vi "MGCC_EnergyMgmt_EMS.vi"() -> ()   [LabVIEW 2016]
uses:
  <vilib>/imath/engines/lvmath2/RunTimeEngine/IndexRead/NIMS V(S).vi
  <vilib>/imath/engines/lvmath2/RunTimeEngine/ErrorHandling/NIMS_Create Error From Enums.vi
  <vilib>/imath/engines/lvmath2/RunTimeEngine/BuiltInFunctions/tril/NIMS_tril.vi
  <vilib>/imath/engines/lvmath2/RunTimeEngine/BuiltInFunctions/double/NIMS_double.vi
  <vilib>/imath/engines/lvmath2/RunTimeEngine/NodeEndStatement/NIMS_NodeEndStatement_Output.vi
  <vilib>/imath/engines/lvmath2/RunTimeEngine/ErrorHandling/NIMS_Finalize Error.vi
  <vilib>/imath/engines/lvmath2/RunTimeEngine/RowToken/NIMS_RowToken_M_CV.vi
  <vilib>/imathl/engines/lvmath/Functions/Error Handling/Create Error.vi
  <vilib>/imath/engines/lvmath/Functions/Error Handling/MergeErrorsWrapper.vi
  <vilib>/imath/engines/lvmath2/RunTimeEngine/IndexRead/NIMS V(R2).vi
  <vilib>/imath/engines/lvmath2/RunTimeEngine/MatrixToken/NIMS_MatrixToken_M_M.vi
  <vilib>/imath/engines/lvmath2/RunTimeEngine/BuiltInFunctions/fmin_lp/NIMS_fmin_lp.vi
  <vilib>/imath/engines/lvmath2/RunTimeEngine/RowToken/NIMS_RowToken_M_M.vi
  <vilib>/imath/engines/lvmath2/RunTimeEngine/BuiltInFunctions/length/NIMS_length(GV).vi
  <vilib>/imath/engines/lvmath2/RunTimeEngine/BuiltInFunctions/eye/NIMS_M=eye(I32).vi
  <vilib>/imath/engines/lvmath2/RunTimeEngine/MatrixToken/NIMS_MatrixToken_M_SorCV.vi
  <vilib>/imath/engines/lvmath2/RunTimeEngine/BuiltInFunctions/is_nan/NIMS_is_nan.vi
  <vilib>/ErrorRing/Error Ring.xnode
  <vilib>/Utility/error.llb/Error Cluster From Error Code.vi
  <vilib>/imath/engines/lvmath2/RunTimeEngine/BuiltInFunctions/max/1 input/NIMS_max(RV).vi
  <vilib>/imath/engines/lvmath2/RunTimeEngine/IndexRead/NIMS V(R3).vi
  <vilib>/imath/engines/lvmath2/RunTimeSupport/NIMS_Get Scalar_w Error.vi
  <vilib>/imath/engines/lvmath2/RunTimeEngine/MatrixToken/NIMS_MatrixToken_M_RV.vi
  <vilib>/imath/engines/lvmath2/RunTimeEngine/BuiltInFunctions/mean/NIMS_RS=mean(RV,I32).vi
  <vilib>/imath/engines/lvmath2/RunTimeEngine/RowToken/NIMS_RowToken_CV_CV.vi
  <vilib>/imath/engines/lvmath2/RunTimeEngine/IndexRead/NIMS M(S,$).vi
  <vilib>/imath/engines/lvmath2/RunTimeEngine/RangeToken/NIMS_Range_R2 - Integer.vi
  <vilib>/imath/engines/lvmath2/RunTimeEngine/ArithmeticOperatorToken/NIMS_ArithmeticOperator_multmx(RV,M)-internal.vi
  <vilib>/imath/engines/lvmath2/RunTimeEngine/BuiltInFunctions/ones/NIMS_V=ones(I32,I32).vi
  <vilib>/imath/engines/lvmath2/RunTimeEngine/ArithmeticOperatorToken/NIMS_ArithmeticOperator_plus.vi
  <vilib>/imath/engines/lvmath2/RunTimeEngine/ArithmeticOperatorToken/NIMS_ArithmeticOperator_minus.vi
  <vilib>/imath/engines/lvmath2/RunTimeEngine/IndexReplace/NIMS V(S)=S.vi
  <vilib>/imath/engines/lvmath2/RunTimeEngine/CommandStatement/MC_CommandStatement_break.vi
  <vilib>/imath/engines/lvmath2/RunTimeEngine/BuiltInFunctions/min/1 input/NIMS_min(RV).vi
  <vilib>/imath/engines/lvmath2/RunTimeEngine/BuiltInFunctions/abs/NIMS_abs(signed).vi
  <vilib>/imath/engines/lvmath2/RunTimeEngine/BuiltInFunctions/findnz/NIMS_[1o]_findnz(GRowV).vi
  <vilib>/imath/engines/lvmath2/RunTimeEngine/BuiltInFunctions/is_empty/NIMS_is_empty(GV).vi
  <vilib>/imath/engines/lvmath2/RunTimeEngine/IndexRead/NIMS M($,V).vi
  <vilib>/imath/engines/lvmath2/RunTimeEngine/IndexReplace/NIMS M($,S)=M.vi
  <vilib>/imath/engines/lvmath2/RunTimeEngine/IndexRead/NIMS M($,S).vi
  <vilib>/imath/engines/lvmath2/RunTimeEngine/ArithmeticOperatorToken/NIMS_ArithmeticOperator_multmx(RV,CV)-internal.vi
panel:
  out "error out ISD1":errorcluster
  out "P_batt1 2":dbl[](array[numeric])
  out "P_batt 3":dbl[](array[numeric])
  out "P_pv1":dbl[](array[numeric])
  out "P_pv":dbl[](array[numeric])
  out "error out 3":errorcluster
  out "L9":dbl[](array[numeric])
  out "L8":dbl[](array[numeric])
  out "L7":dbl[](array[numeric])
  out "L5":dbl[](array[numeric])
  out "L4":dbl[](array[numeric])
  out "L3":dbl[](array[numeric])
  out "L2":dbl[](array[numeric])
  out "L11":dbl[](array[numeric])
  out "L10":dbl[](array[numeric])
  out "P_batt1":dbl[](array[numeric])
  out "HIS8":dbl[](array[numeric])
  out "HIS7":dbl[](array[numeric])
  out "HIS5":dbl[](array[numeric])
  out "HIS4":dbl[](array[numeric])
  out "HIS3":dbl[](array[numeric])
  out "HIS2":dbl[](array[numeric])
  out "HIS9":dbl[](array[numeric])
  out "HIS11":dbl[](array[numeric])
  out "HIS10":dbl[](array[numeric])
  out "P_batt 2":dbl[](array[numeric])
  out "f_MGCC_PVFcst_FcstPV 2":dbl[](array[numeric])
  out "BESS-SOC 2":dbl
  out "Ld 2":dbl[](array[numeric])
  out "error out 2":errorcluster
  out "P_batt":dbl[](array[numeric])
  out "f_MGCC_PVFcst_FcstPV":dbl[](array[numeric])
  out "BESS-SOC":dbl
  out "Ld":dbl[](array[numeric])
  out "error out":errorcluster
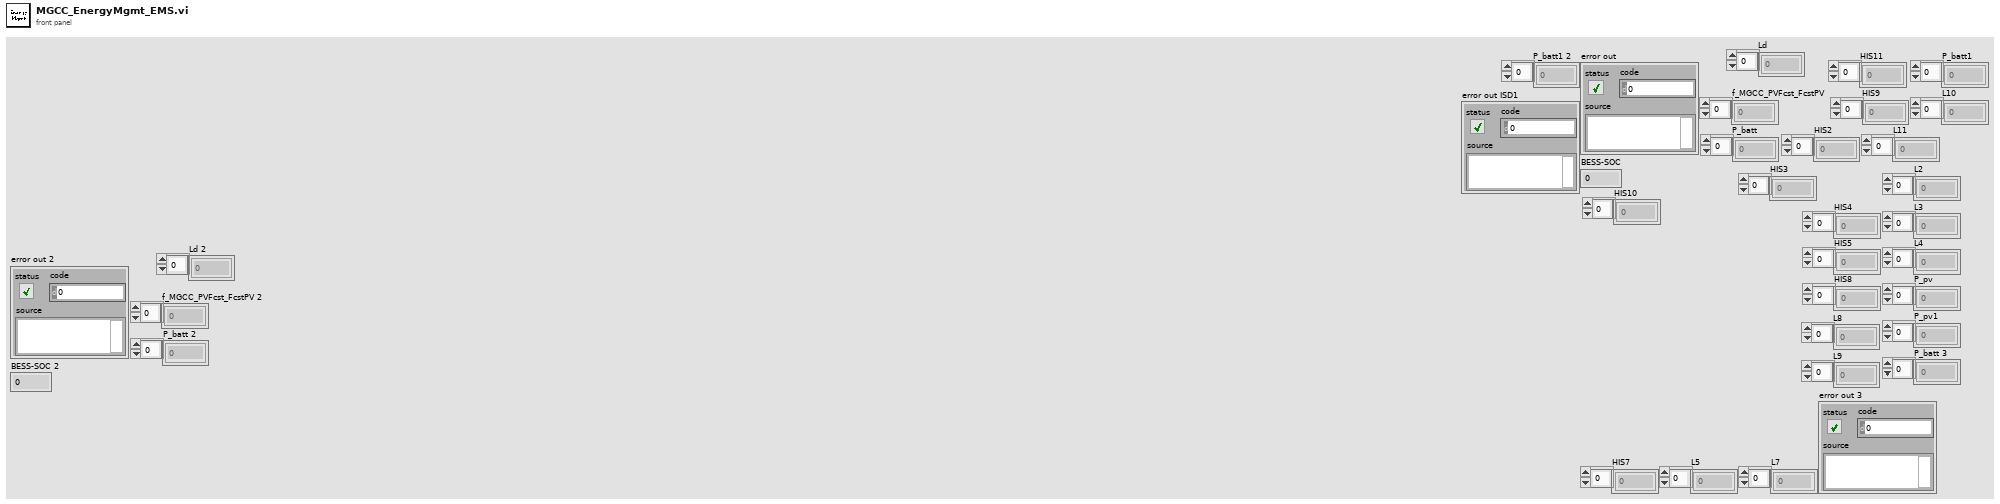
[diagram p1: front panel]
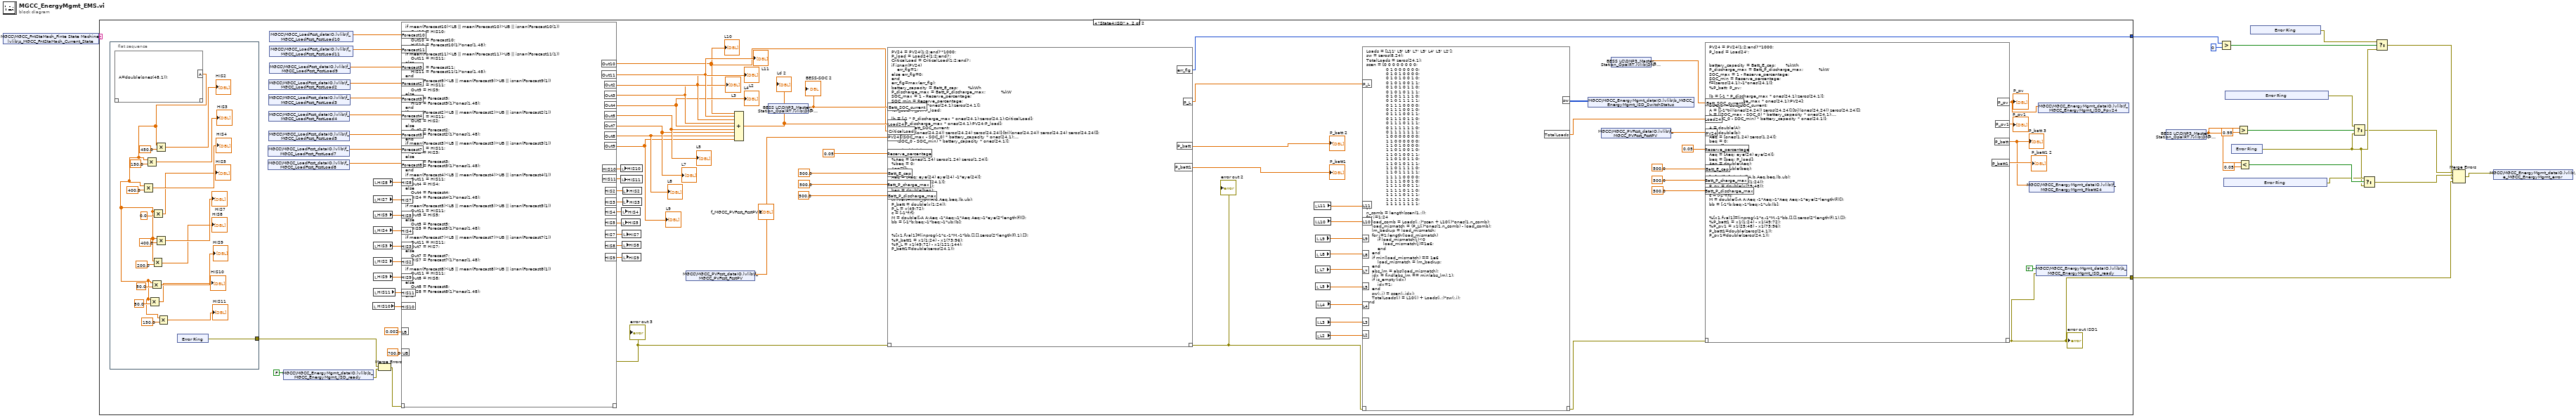
[diagram p0: block diagram]
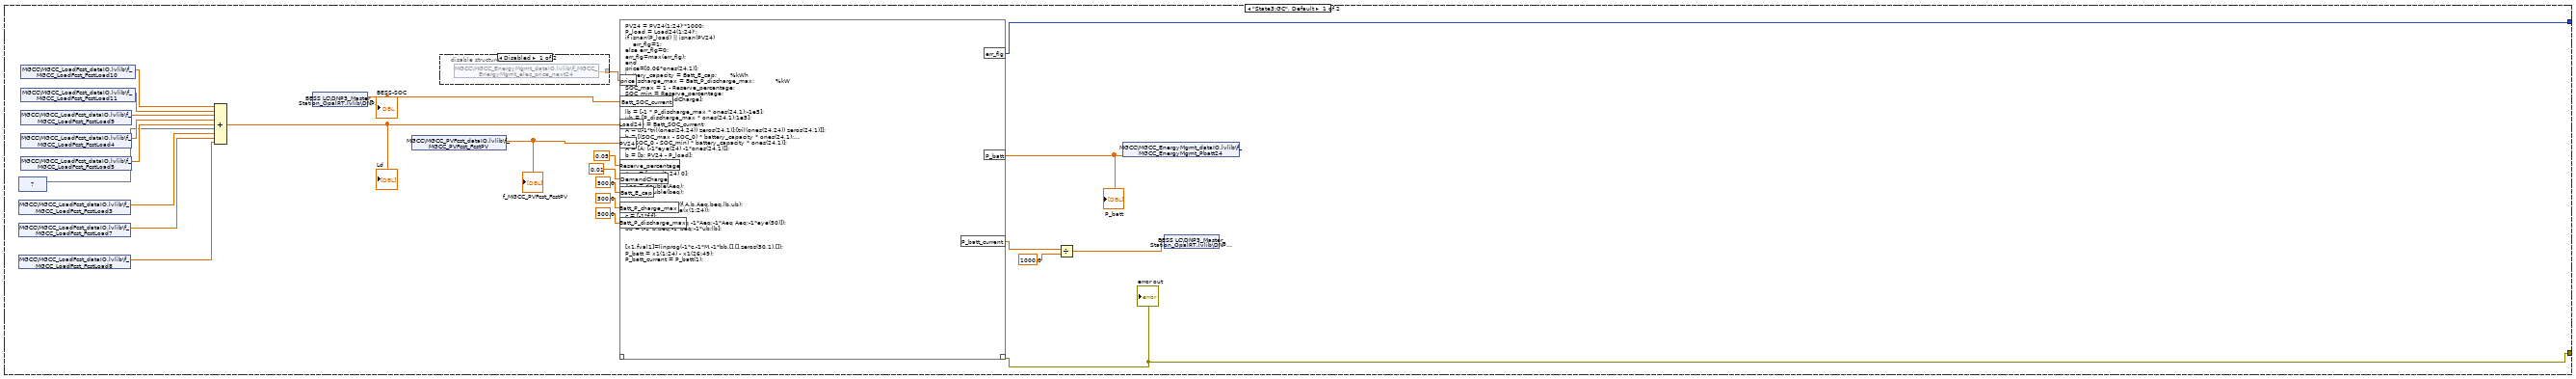
[diagram p2: hidden frame]
diagram:
  n1 = shared-variable "MGCC\\MGCC_FntStaMach_Finte State Machine.lvlib\\s_MGCC_FntStaMach_Current_State"() -> (w18:string)  [unwired: 1 in, 1 out]
  n2 = case shown="\"State4:ISD\"" w18 {
    tunnel: [w20 w529] -> w9
    tunnel: [w19 w528] -> w2
    frame "State3:GC", Default {
      n3 = shared-variable "?"() -> (w27)  [unwired: 1 in, 1 out]
      n4 = shared-variable "MGCC\\MGCC_LoadFcst_dataIO.lvlib\\f_MGCC_LoadFcst_FcstLoad3"() -> (w24:dbl[])  [unwired: 1 in, 1 out]
      n5 = shared-variable "MGCC\\MGCC_LoadFcst_dataIO.lvlib\\f_MGCC_LoadFcst_FcstLoad7"() -> (w25:dbl[])  [unwired: 1 in, 1 out]
      n6 = shared-variable "MGCC\\MGCC_LoadFcst_dataIO.lvlib\\f_MGCC_LoadFcst_FcstLoad8"() -> (w26:dbl[])  [unwired: 1 in, 1 out]
      n7 = shared-variable "MGCC\\MGCC_LoadFcst_dataIO.lvlib\\f_MGCC_LoadFcst_FcstLoad10"() -> (w35:dbl[])  [unwired: 1 in, 1 out]
      n8 = shared-variable "MGCC\\MGCC_LoadFcst_dataIO.lvlib\\f_MGCC_LoadFcst_FcstLoad11"() -> (w34:dbl[])  [unwired: 1 in, 1 out]
      n9 = shared-variable "MGCC\\MGCC_LoadFcst_dataIO.lvlib\\f_MGCC_LoadFcst_FcstLoad9"() -> (w33:dbl[])  [unwired: 1 in, 1 out]
      n10 = shared-variable "MGCC\\MGCC_LoadFcst_dataIO.lvlib\\f_MGCC_LoadFcst_FcstLoad4"() -> (w32:dbl[])  [unwired: 1 in, 1 out]
      n11 = shared-variable "MGCC\\MGCC_LoadFcst_dataIO.lvlib\\f_MGCC_LoadFcst_FcstLoad5"() -> (w31:dbl[])  [unwired: 1 in, 1 out]
      n12 = Compound Arithmetic op=ADD(w35, w34, w33, w32, w31, w27, w24, w25, w26) -> (w30:dbl[])
      "Ld" <- w30
      n13 = shared-variable "BESS LC\\DNP3_Master_Station_OpalRT.lvlib\\DNP3_Master_Data_Variables.lvlib\\MS_Analog_Status.lvlib\\BESS-SOC"() -> (w28:dbl)  [unwired: 1 in, 1 out]
      "BESS-SOC" <- w28
      n14 = shared-variable "MGCC\\MGCC_PVFcst_dataIO.lvlib\\f_MGCC_PVFcst_FcstPV"() -> (w37:dbl[])  [unwired: 1 in, 1 out]
      "f_MGCC_PVFcst_FcstPV" <- w37
      n15 = disable-structure shown="Disabled" {
        disable-tunnel: [w43 _] -> w42
        frame Disabled {
          n16 = shared-variable "MGCC\\MGCC_EnergyMgmt_dataIO.lvlib\\f_MGCC_EnergyMgmt_elec_price_next24"() -> (w43:dbl[])  [unwired: 1 in, 1 out]
        }
        frame Enabled {
        }
      }
      n17 = mathscript code="PV24 = PV24(1:24)'*1000;\nP_load = Load24(1:24)';\nif isnan(P_load) || isnan(PV24)\n    err_flg=1;\nelse err_flg=0;\nerr_flg=max(err_flg);\nend\nprice=[0.06*ones(24,1)];\nbattery_capacity = Batt_E_cap;       %kWh\nP_discharge_max = Batt_P_discharge_max;           %kW\nSOC_max = 1 - Reserve_percentage;\nSOC_min = Reserve_percentage;\nf=[-price;DemandCharge];\n\nlb = [-1 * P_discharge_max * ones(24,1);-1e5];\nub = [P_discharge_max * ones(24,1);1e5];\nSOC_0 = Batt_SOC_current;\nA = [[-1*tril(ones(24,24)) zeros(24,1)];[tril(ones(24,24)) zeros(24,1)]];\nb = [(SOC_max - SOC_0) * battery_capacity * ones(24,1);...\n    (SOC_0 - SOC_min) * battery_capacity * ones(24,1)];\nA = [A; [-1*eye(24) -1*ones(24,1)]];\nb = [b; PV24 - P_load];\nA = double(A);\nb = double(b);\nAeq = [ones(1,24) 0];\nbeq = 0;\nAeq = double(Aeq);\nbeq = double(beq);\n\n%[x,fval]=fmin_lp(f,A,b,Aeq,beq,lb,ub);\n%P_batt1 = double(x(1:24));\nc = [-1*f;f];\nM = double([-A A;Aeq -1*Aeq;-1*Aeq Aeq;-1*eye(50)]);\nbb = [-1*b;beq;-1*beq;-1*ub;lb];\n\n\n[x1,fval1]=linprog(-1*c,-1*M,-1*bb,[],[],zeros(50,1),[]);\nP_batt = x1(1:24) - x1(26:49);\nP_batt_current = P_batt(1);"("price"=w42, "Batt_E_cap"=500.0, "Batt_P_charge_max"=500.0, "Batt_P_discharge_max"=500.0, "Batt_SOC_current"=w28, "DemandCharge"=0.01, "Load24"=w30, "PV24"=w37, "Reserve_percentage"=0.05) -> ("??"=w19:errorcluster, "P_batt"=w29:dbl[], "P_batt_current"=w22:dbl, "err_flg"=w20:i32)  [unwired: 1 in]
      "error out" <- w19
      "P_batt" <- w29
      n18 = Divide(x=w22, y=1000.0) -> (x/y=w23:dbl)
      n19 = shared-variable "MGCC\\MGCC_EnergyMgmt_dataIO.lvlib\\f_MGCC_EnergyMgmt_Pbatt24"(w29) -> ()  [unwired: 1 in, 1 out]
      n20 = shared-variable "BESS LC\\DNP3_Master_Station_OpalRT.lvlib\\DNP3_Master_Data_Variables.lvlib\\MS_Analog_Control.lvlib\\BESS-APC"(w23) -> ()  [unwired: 1 in, 1 out]
    }
    frame "State4:ISD" {
      n21 = flat-sequence {
        tunnel: [w623] -> w525
        frame #0 {
          n22 = mathscript code="A=double(ones(48,1));"() -> ("A"=w605:dbl[])  [unwired: 1 in, 1 out]
          n23 = Multiply(x=w605, y=400.0) -> (x*y=→"HIS4":dbl[])
          n24 = Multiply(x=w605, y=150.0) -> (x*y=→"HIS3":dbl[])
          n25 = Multiply(x=w605, y=50.0) -> (x*y=→"HIS10":dbl[])
          n26 = Multiply(x=w605, y=50.0) -> (x*y=→"HIS9":dbl[])
          n27 = Multiply(x=w605, y=200.0) -> (x*y=→"HIS8":dbl[])
          n28 = Multiply(x=w605, y=0.0) -> (x*y=→"HIS5":dbl[])
          n29 = Multiply(x=w605, y=450.0) -> (x*y=→"HIS2":dbl[])
          n30 = Multiply(x=w605, y=400.0) -> (x*y=→"HIS7":dbl[])
          n31 = Multiply(x=w605, y=150.0) -> (x*y=→"HIS11":dbl[])
          n32 = xnode "Error Ring"() -> ("error out"=w623:errorcluster)
        }
      }
      n33 = shared-variable "MGCC\\MGCC_LoadFcst_dataIO.lvlib\\f_MGCC_LoadFcst_FcstLoad7"() -> (w588:dbl[])  [unwired: 1 in, 1 out]
      n34 = shared-variable "MGCC\\MGCC_LoadFcst_dataIO.lvlib\\f_MGCC_LoadFcst_FcstLoad8"() -> (w587:dbl[])  [unwired: 1 in, 1 out]
      n35 = shared-variable "MGCC\\MGCC_LoadFcst_dataIO.lvlib\\f_MGCC_LoadFcst_FcstLoad4"() -> (w590:dbl[])  [unwired: 1 in, 1 out]
      n36 = shared-variable "MGCC\\MGCC_LoadFcst_dataIO.lvlib\\f_MGCC_LoadFcst_FcstLoad5"() -> (w589:dbl[])  [unwired: 1 in, 1 out]
      n37 = shared-variable "MGCC\\MGCC_LoadFcst_dataIO.lvlib\\f_MGCC_LoadFcst_FcstLoad2"() -> (w592:dbl[])  [unwired: 1 in, 1 out]
      n38 = shared-variable "MGCC\\MGCC_LoadFcst_dataIO.lvlib\\f_MGCC_LoadFcst_FcstLoad3"() -> (w591:dbl[])  [unwired: 1 in, 1 out]
      n39 = shared-variable "MGCC\\MGCC_LoadFcst_dataIO.lvlib\\f_MGCC_LoadFcst_FcstLoad10"() -> (w595:dbl[])  [unwired: 1 in, 1 out]
      n40 = shared-variable "MGCC\\MGCC_LoadFcst_dataIO.lvlib\\f_MGCC_LoadFcst_FcstLoad11"() -> (w594:dbl[])  [unwired: 1 in, 1 out]
      n41 = shared-variable "MGCC\\MGCC_LoadFcst_dataIO.lvlib\\f_MGCC_LoadFcst_FcstLoad9"() -> (w593:dbl[])  [unwired: 1 in, 1 out]
      n42 = shared-variable "MGCC\\MGCC_EnergyMgmt_dataIO.lvlib\\b_MGCC_EnergyMgmt_ISD_ready"(FALSE ("b_MGCC_EnergyMgmt_ISD_ready")) -> (error out=w526:errorcluster)  [unwired: 1 in]
      n43 = local read "HIS10"() -> (w578:dbl[])
      n44 = local read "HIS8"() -> (w586:dbl[])
      n45 = local read "HIS7"() -> (w585:dbl[])
      n46 = local read "HIS5"() -> (w584:dbl[])
      n47 = local read "HIS4"() -> (w583:dbl[])
      n48 = local read "HIS3"() -> (w582:dbl[])
      n49 = local read "HIS2"() -> (w581:dbl[])
      n50 = local read "HIS9"() -> (w580:dbl[])
      n51 = local read "HIS11"() -> (w579:dbl[])
      n52 = Merge Errors(w525, w526) -> (w527:errorcluster)
      n53 = mathscript code="if mean(Forecast10)<LB || mean(Forecast10)>UB || isnan(Forecast10(1))\n    Out10 = HIS10;\nelse\n    Out10 = Forecast10;\n    HIS10 = Forecast10(1)*ones(1,48);\nend\nif mean(Forecast11)<LB || mean(Forecast11)>UB || isnan(Forecast11(1))\n    Out11 = HIS11;\nelse\n    Out11 = Forecast11;\n    HIS11 = Forecast11(1)*ones(1,48);\nend\nif mean(Forecast9)<LB || mean(Forecast9)>UB || isnan(Forecast9(1))\n    Out11 = HIS11;\n    Out9 = HIS9;\nelse\n    Out9 = Forecast9;\n    HIS9 = Forecast9(1)*ones(1,48);\nend\nif mean(Forecast2)<LB || mean(Forecast2)>UB || isnan(Forecast2(1))\n    Out11 = HIS11;\n    Out2 = HIS2;\nelse\n    Out2 = Forecast2;\n    HIS2 = Forecast2(1)*ones(1,48);\nend\nif mean(Forecast3)<LB || mean(Forecast3)>UB || isnan(Forecast3(1))\n    Out11 = HIS11;\n    Out3 = HIS3;\nelse\n    Out3 = Forecast3;\n    HIS3 = Forecast3(1)*ones(1,48);\nend\nif mean(Forecast4)<LB || mean(Forecast4)>UB || isnan(Forecast4(1))\n    Out11 = HIS11;\n    Out4 = HIS4;\nelse\n    Out4 = Forecast4;\n    HIS4 = Forecast4(1)*ones(1,48);\nend\nif mean(Forecast5)<LB || mean(Forecast5)>UB || isnan(Forecast5(1))\n    Out11 = HIS11;\n    Out5 = HIS5;\nelse\n    Out5 = Forecast5;\n    HIS5 = Forecast5(1)*ones(1,48);\nend\nif mean(Forecast7)<LB || mean(Forecast7)>UB || isnan(Forecast7(1))\n    Out11 = HIS11;\n    Out7 = HIS7;\nelse\n    Out7 = Forecast7;\n    HIS7 = Forecast7(1)*ones(1,48);\nend\nif mean(Forecast8)<LB || mean(Forecast8)>UB || isnan(Forecast8(1))\n    Out11 = HIS11;\n    Out8 = HIS8;\nelse\n    Out8 = Forecast8;\n    HIS8 = Forecast8(1)*ones(1,48);\nend"("??"=w527, "Forecast10"=w595, "Forecast11"=w594, "Forecast9"=w593, "Forecast2"=w592, "Forecast3"=w591, "Forecast4"=w590, "Forecast5"=w589, "Forecast7"=w588, "Forecast8"=w587, "HIS8"=w586, "HIS7"=w585, "HIS5"=w584, "HIS4"=w583, "HIS3"=w582, "HIS2"=w581, "HIS9"=w580, "HIS11"=w579, "HIS10"=w578, "LB"=0.002, "UB"=700.0) -> ("??"=w557:errorcluster, "Out10"=w534:dbl[], "HIS10"=w575:dbl[], "HIS11"=w574:dbl[], "HIS2"=w573:dbl[], "HIS3"=w572:dbl[], "HIS4"=w571:dbl[], "HIS5"=w570:dbl[], "HIS7"=w569:dbl[], "HIS8"=w568:dbl[], "HIS9"=w567:dbl[], "Out11"=w566:dbl[], "Out2"=w565:dbl[], "Out3"=w564:dbl[], "Out4"=w563:dbl[], "Out5"=w562:dbl[], "Out7"=w561:dbl[], "Out8"=w560:dbl[], "Out9"=w559:dbl[])
      "L10" <- w534
      "L11" <- w566
      "L2" <- w565
      "L3" <- w564
      "L4" <- w563
      "L5" <- w562
      "L7" <- w561
      "L8" <- w560
      "L9" <- w559
      "error out 3" <- w557
      n54 = local write "HIS10"(w575) -> ()
      n55 = local write "HIS11"(w574) -> ()
      n56 = local write "HIS4"(w571) -> ()
      n57 = local write "HIS5"(w570) -> ()
      n58 = local write "HIS7"(w569) -> ()
      n59 = local write "HIS8"(w568) -> ()
      n60 = local write "HIS9"(w567) -> ()
      n61 = local write "HIS2"(w573) -> ()
      n62 = local write "HIS3"(w572) -> ()
      n63 = shared-variable "MGCC\\MGCC_PVFcst_dataIO.lvlib\\f_MGCC_PVFcst_FcstPV"() -> (w600:dbl[])  [unwired: 1 in, 1 out]
      "f_MGCC_PVFcst_FcstPV 2" <- w600
      n64 = Compound Arithmetic op=ADD(w534, w566, w565, w564, w563, w562, w561, w560, w559) -> (w598:dbl[])
      "Ld 2" <- w598
      n65 = shared-variable "BESS LC\\DNP3_Master_Station_OpalRT.lvlib\\DNP3_Master_Data_Variables.lvlib\\MS_Analog_Status.lvlib\\BESS-SOC"() -> (w596:dbl)  [unwired: 1 in, 1 out]
      "BESS-SOC 2" <- w596
      n66 = mathscript code="PV24 = PV24(1:2:end)'*1000;\nP_load = Load24(1:2:end)';\nCriticalLoad = CriticalLoad(1:2:end)';\nif isnan(PV24)\n    err_flg=1;\nelse err_flg=0;\nend\nerr_flg=max(err_flg);\nbattery_capacity = Batt_E_cap;       %kWh\nP_discharge_max = Batt_P_discharge_max;           %kW\nSOC_max = 1 - Reserve_percentage;\nSOC_min = Reserve_percentage;\nf=[zeros(24,1);-1*ones(24,1);zeros(24,1)];\n%P_batt; P_pv; P_load;\n\nlb = [-1 * P_discharge_max * ones(24,1);zeros(24,1);CriticalLoad];\nub = [P_discharge_max * ones(24,1);PV24;P_load];\nSOC_0 = Batt_SOC_current;\nA = [[-1*tril(ones(24,24)) zeros(24,24) zeros(24,24)];[tril(ones(24,24)) zeros(24,24) zeros(24,24)]];\nb = [(SOC_max - SOC_0) * battery_capacity * ones(24,1);...\n    (SOC_0 - SOC_min) * battery_capacity * ones(24,1)];\n\nA = double(A);\nb = double(b);\n%Aeq = [ones(1,24) zeros(1,24) zeros(1,24)];\n%beq = 0;\nAeq=[];\nbeq=[];\nAeq = [Aeq; eye(24) eye(24) -1*eye(24)];\nbeq = [beq; zeros(24,1)];\nAeq = double(Aeq);\nbeq = double(beq);\n\n[x,fval]=fmin_lp(f,A,b,Aeq,beq,lb,ub);\nP_batt = double(x(1:24));\nP_L = x(49:72);\nc = [-1*f;f];\nM = double([-A A;Aeq -1*Aeq;-1*Aeq Aeq;-1*eye(2*length(f))]);\nbb = [-1*b;beq;-1*beq;-1*ub;lb];\n\n\n%[x1,fval1]=linprog(-1*c,-1*M,-1*bb,[],[],zeros(2*length(f),1),[]);\n%P_batt1 = x1(1:24) - x1(73:96);\n%P_L = x1(49:72) - x1(121:144);\nP_batt1=double(zeros(24,1));"("??"=w557, "Batt_E_cap"=500.0, "Batt_P_charge_max"=500.0, "Batt_P_discharge_max"=500.0, "Batt_SOC_current"=w596, "Load24"=w598, "PV24"=w600, "Reserve_percentage"=0.05, "CriticalLoad"=w534) -> ("??"=w546:errorcluster, "P_batt"=→"P_batt 2":dbl[], "P_batt1"=→"P_batt1":dbl[], "P_L"=w556:dbl[], "err_flg"=w529:i32)
      "error out 2" <- w546
      n67 = local read "L11"() -> (w555:dbl[])
      n68 = local read "L10"() -> (w554:dbl[])
      n69 = local read "L9"() -> (w553:dbl[])
      n70 = local read "L8"() -> (w552:dbl[])
      n71 = local read "L7"() -> (w551:dbl[])
      n72 = local read "L5"() -> (w550:dbl[])
      n73 = local read "L4"() -> (w549:dbl[])
      n74 = local read "L3"() -> (w548:dbl[])
      n75 = local read "L2"() -> (w547:dbl[])
      n76 = mathscript code="Loads = [L11' L9' L8' L7' L5' L4' L3' L2'];\nsw = zeros(8,24);\nTotalLoads = zeros(24,1);\nscen = [0 0 0 0 0 0 0 0;\n              0 1 0 0 0 0 0 0;\n              0 1 0 1 0 0 0 0;\n              0 1 0 1 0 0 1 0;\n              0 1 0 1 0 0 1 1;\n              0 1 0 1 0 1 1 0;\n              0 1 0 1 0 1 1 1;\n              0 1 0 1 1 1 1 0;\n              0 1 0 1 1 1 1 1;\n              0 1 1 1 0 0 0 0;\n              0 1 1 1 0 0 1 0;\n              0 1 1 1 0 0 1 1;\n              0 1 1 1 0 1 1 0;\n              0 1 1 1 0 1 1 1;\n              0 1 1 1 1 1 1 0;\n              0 1 1 1 1 1 1 1;\n              1 0 0 0 0 0 0 0;\n              1 1 0 0 0 0 0 0;\n              1 1 0 1 0 0 0 0;\n              1 1 0 1 0 0 1 0;\n              1 1 0 1 0 0 1 1;\n              1 1 0 1 0 1 1 0;\n              1 1 0 1 0 1 1 1;\n              1 1 0 1 1 1 1 0;\n              1 1 0 1 1 1 1 1;\n              1 1 1 1 0 0 0 0;\n              1 1 1 1 0 0 1 0;\n              1 1 1 1 0 0 1 1;\n              1 1 1 1 0 1 1 0;\n              1 1 1 1 0 1 1 1;\n              1 1 1 1 1 1 1 0;\n              1 1 1 1 1 1 1 1;\n]';\nn_comb = length(scen(1,:));\nfor i=1:24\n    load_comb = Loads(i,:)*scen + L10(i)*ones(1,n_comb);\n    load_mismatch = (P_L(i)*ones(1,n_comb) - load_comb);\n    lm_backup = load_mismatch;\n    for j=1:length(load_mismatch)\n        if load_mismatch(j)<0\n            load_mismatch(j)=1e6;\n        end\n    end\n    if min(load_mismatch) == 1e6\n        load_mismatch = lm_backup;\n    end\n    abs_lm = abs(load_mismatch);\n    idx = find(abs_lm == min(abs_lm),1);\n    if is_empty(idx)\n        idx=1;\n    end\n    sw(:,i) = scen(:,idx);\n    TotalLoads(i) = L10(i) + Loads(i,:)*sw(:,i);\nend"("??"=w546, "P_L"=w556, "L11"=w555, "L10"=w554, "L9"=w553, "L8"=w552, "L7"=w551, "L5"=w550, "L4"=w549, "L3"=w548, "L2"=w547) -> ("??"=w537:errorcluster, "sw"=w545:i32[][], "TotalLoads"=w539:dbl[])
      n77 = shared-variable "MGCC\\MGCC_EnergyMgmt_dataIO.lvlib\\b_MGCC_EnergyMgmt_ISD_SwitchStatus"(w545) -> ()  [unwired: 1 in, 1 out]
      n78 = shared-variable "MGCC\\MGCC_PVFcst_dataIO.lvlib\\f_MGCC_PVFcst_FcstPV"() -> (w538:dbl[])  [unwired: 1 in, 1 out]
      n79 = shared-variable "BESS LC\\DNP3_Master_Station_OpalRT.lvlib\\DNP3_Master_Data_Variables.lvlib\\MS_Analog_Status.lvlib\\BESS-SOC"() -> (w540:dbl)  [unwired: 1 in, 1 out]
      n80 = mathscript code="PV24 = PV24(1:2:end)'*1000;\nP_load = Load24';\n\n\nbattery_capacity = Batt_E_cap;       %kWh\nP_discharge_max = Batt_P_discharge_max;           %kW\nSOC_max = 1 - Reserve_percentage;\nSOC_min = Reserve_percentage;\nf=[zeros(24,1);-1*ones(24,1)];\n%P_batt; P_pv; \n\nlb = [-1 * P_discharge_max * ones(24,1);zeros(24,1)];\nub = [P_discharge_max * ones(24,1);PV24];\nSOC_0 = Batt_SOC_current;\nA = [[-1*tril(ones(24,24)) zeros(24,24)];[tril(ones(24,24)) zeros(24,24)]];\nb = [(SOC_max - SOC_0) * battery_capacity * ones(24,1);...\n    (SOC_0 - SOC_min) * battery_capacity * ones(24,1)];\n\nA = double(A);\nb = double(b);\nAeq = [ones(1,24) zeros(1,24)];\nbeq = 0;\nAeq=[];\nbeq=[];\nAeq = [Aeq; eye(24) eye(24)];\nbeq = [beq; P_load];\nAeq = double(Aeq);\nbeq = double(beq);\n\n[x,fval]=fmin_lp(f,A,b,Aeq,beq,lb,ub);\nP_batt = double(x(1:24));\nP_pv = double(x(25:48));\n\nc = [-1*f;f];\nM = double([-A A;Aeq -1*Aeq;-1*Aeq Aeq;-1*eye(2*length(f))]);\nbb = [-1*b;beq;-1*beq;-1*ub;lb];\n\n\n%[x1,fval1]=linprog(-1*c,-1*M,-1*bb,[],[],zeros(2*length(f),1),[]);\n%P_batt1 = x1(1:24) - x1(49:72);\n%P_pv1 = x1(25:48) - x1(73:96);\nP_batt1=double(zeros(24,1));\nP_pv1=double(zeros(24,1));"("??"=w537, "Batt_E_cap"=500.0, "Batt_P_charge_max"=500.0, "Batt_P_discharge_max"=500.0, "Batt_SOC_current"=w540, "Load24"=w539, "PV24"=w538, "Reserve_percentage"=0.05) -> ("??"=w528:errorcluster, "P_batt"=w532:dbl[], "P_batt1"=→"P_batt1 2":dbl[], "P_pv"=w531:dbl[], "P_pv1"=→"P_pv1":dbl[])
      "P_pv" <- w531
      "P_batt 3" <- w532
      "error out ISD1" <- w528
      n81 = shared-variable "MGCC\\MGCC_EnergyMgmt_dataIO.lvlib\\f_MGCC_EnergyMgmt_Pbatt24"(w532) -> ()  [unwired: 1 in, 1 out]
      n82 = shared-variable "MGCC\\MGCC_EnergyMgmt_dataIO.lvlib\\b_MGCC_EnergyMgmt_ISD_ready"(TRUE ("b_MGCC_EnergyMgmt_ISD_ready"), error in=w528) -> ()  [unwired: 1 out]
      n83 = shared-variable "MGCC\\MGCC_EnergyMgmt_dataIO.lvlib\\f_MGCC_EnergyMgmt_ISD_Ppv24"(w531) -> ()  [unwired: 1 in, 1 out]
    }
  }
  n84 = shared-variable "BESS LC\\DNP3_Master_Station_OpalRT.lvlib\\DNP3_Master_Data_Variables.lvlib\\MS_Analog_Status.lvlib\\BESS-SOC"() -> (w17:dbl)  [unwired: 1 in, 1 out]
  n85 = Greater?(x=w9, y=0) -> (0:w8:bool)
  n86 = xnode "Error Ring"() -> ("error out"=w11:errorcluster)
  n87 = xnode "Error Ring"() -> ("error out"=w13:errorcluster)
  n88 = xnode "Error Ring"() -> ("error out"=w6:errorcluster)
  n89 = Greater?(x=w17, y=0.95) -> (0:w14:bool)
  n90 = Less?(x=w17, y=0.05) -> (x < y?=w12:bool)
  n91 = xnode "Error Ring"() -> ("error out"=w7:errorcluster)
  n92 = Select(t=w13, s=w14, f=w6) -> (s? t:f=w5:errorcluster)
  n93 = Select(t=w11, s=w12, f=w6) -> (s? t:f=w4:errorcluster)
  n94 = Select(t=w7, s=w8, f=w6) -> (s? t:f=w3:errorcluster)
  n95 = Merge Errors(w5, w4, w3, w2) -> (w1:errorcluster)
  n96 = shared-variable "MGCC\\MGCC_EnergyMgmt_dataIO.lvlib\\e_MGCC_EnergyMgmt_error"(w1) -> ()  [unwired: 1 in, 1 out]
